vi "Meacurrent8341.vi"(8 "error in":errorcluster caption="错误输入", 10 "测试类型":u16(ring) items=["DCV", "ACV", "DCI", "ACI", "OHM", "RST", "CAP", "FRQ", "AUTO"], 11 "VISA资源名称":refnum<visa-resource-name>="COM1") -> (0 "错误输出":errorcluster, 2 "数值":dbl format="%#_3g", 3 "响应":string)   [LabVIEW 2013]
uses:
  C:/Program Files/National Instruments/LabVIEW 2013/examples/Instrument IO/Serial/support/Serial - Settings.ctl
  <vilib>/Instr/_visa.llb/VISA Flush IO Buffer Mask.ctl
  <vilib>/Instr/_visa.llb/VISA Configure Serial Port (Instr).vi
panel:
  in  "串口设置":T1={"波特率"=9600, "数据比特"=8, "奇偶"=enum."None", "停止位"=10, "流控制"=0} {"流控制" items=["无"=0, "XON/XOFF"=1, "RTS/CTS"=2, "DTR/DSR"=4]; "停止位" items=["1.0"=10, "1.5"=15, "2.0"=20]; "数据比特" min=5 max=8 step=1; "波特率" items=["75"=75, "110"=110, "134"=134, "150"=150, "300"=300, "600"=600, "1200"=1200, "1800"=1800, "2400"=2400, "4800"=4800, "7200"=7200, "9600"=9600, "14400"=14400, "19200"=19200, "28800"=28800, "38400"=38400, "56000"=56000, "57600"=57600, "115200"=115200, "128000"=128000, "230400"=230400]}
  in  "读取前延时(ms)":u32=200
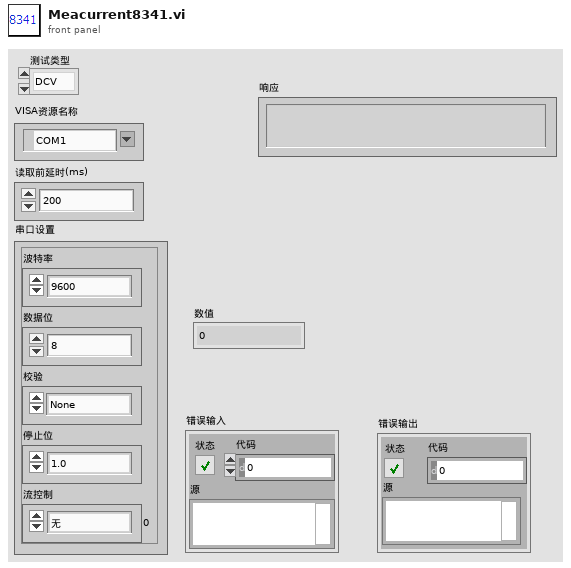
[diagram p1: front panel]
types:
  T1 = typedef "Serial - Settings.ctl" = cluster{"波特率":u32, "数据比特":u16, "奇偶":enum16{"None", "Odd", "Even", "Mark", "Space"}, "停止位":u16, "流控制":u16}
  T2 = typedef "VISA Flush IO Buffer Mask.ctl" = u16
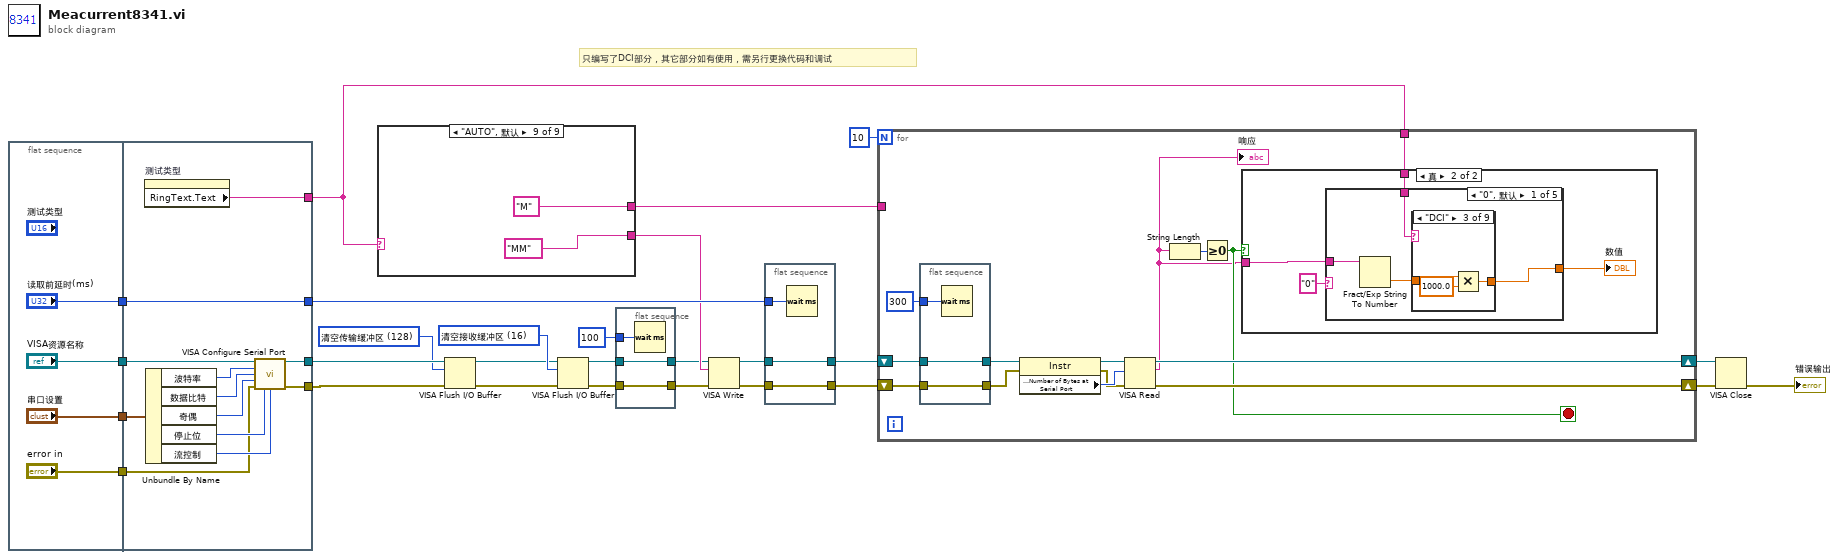
[diagram p0: block diagram]
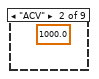
[diagram p4: hidden frame]
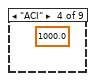
[diagram p5: hidden frame]
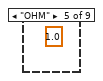
[diagram p6: hidden frame]
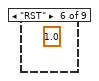
[diagram p7: hidden frame]
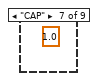
[diagram p8: hidden frame]
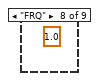
[diagram p9: hidden frame]
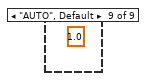
[diagram p10: hidden frame]
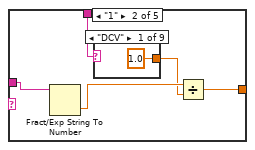
[diagram p11: hidden frame]
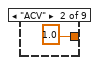
[diagram p12: hidden frame]
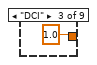
[diagram p13: hidden frame]
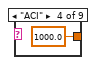
[diagram p14: hidden frame]
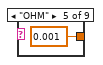
[diagram p15: hidden frame]
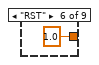
[diagram p16: hidden frame]
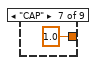
[diagram p17: hidden frame]
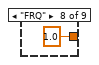
[diagram p18: hidden frame]
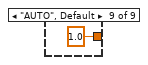
[diagram p19: hidden frame]
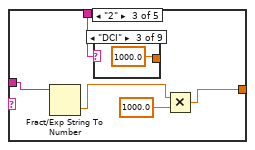
[diagram p20: hidden frame]
diagram:
  w7 = T2 128 items=["清空接收缓冲区"=16, "向设备写入传输缓冲区"=32, "清空接收缓冲区（无I/O）"=64, "清空传输缓冲区"=128] ("Mask")
  w16 = T2 16 items=["清空接收缓冲区"=16, "向设备写入传输缓冲区"=32, "清空接收缓冲区（无I/O）"=64, "清空传输缓冲区"=128] ("Mask")
  # "只编写了DCI部分，其它部分如有使用，需另行更换代码和调试"
  n1 = flat-sequence {
    tunnel: ["VISA资源名称"] -> w15
    tunnel: ["读取前延时(ms)"] -> w14
    tunnel: ["串口设置"] -> w13
    tunnel: ["error in"] -> w1
    tunnel: [w43] -> w23
    tunnel: w15 -> [w36]
    tunnel: w14 -> [w43]
    tunnel: w13 -> [w37]
    tunnel: [w35] -> w12
    tunnel: [w34] -> w11
    tunnel: [w33] -> w10
    tunnel: w1 -> [w32]
    frame #0 {
    }
    frame #1 {
      n2 = property on="测试类型" class="Ring (严格)"() -> ("RingText.Text"=w33:string)  [unwired: 2 in, 2 out]
      n3 = Unbundle By Name(w37) -> ("波特率"=w38:u32, "数据比特"=w39:u16, "奇偶"=w40:enum16{"None", "Odd", "Even", "Mark", "Space"}, "停止位"=w41:u16, "流控制"=w42:u16)
      n4 = call-poly "VISA Configure Serial Port"("VISA resource name"=w36, "baud rate (9600)"=w38, "data bits (8)"=w39, "parity (0:none)"=w40, "error in (no error)"=w32, "stop bits (10: 1 bit)"=w41, "flow control (0:none)"=w42) -> ("VISA resource name out"=w35:refnum<visa-resource-name>, "error out"=w34:errorcluster)  [unwired: 2 in, 5 out]
    }
  }
  n5 = case shown="\"AUTO\", 默认" w10 {
    tunnel: ["MEAS:VOLT:DC? 50e\n" "MEAS:VOLT:AC? 50e\n" "MEAS:CURR:DC? 5e\n" "MEAS:CURR:AC? 5e\n" "EE" ("Command") "FF" ("Command") "GG" ("Command") "HH" ("Command") "MM" ("Command")] -> w22
    tunnel: ["0" ("Command") "1" ("Command") "3" ("Command") "4" ("Command") "6" ("Command") "F" ("Command") "7" ("Command") "8" ("Command") "M" ("Command")] -> w21
    frame "DCV" {
      n6 = local write "数值"(0.0 ("数值")) -> ()
    }
    frame "ACV" {
      n7 = local write "数值"(0.0 ("数值")) -> ()
    }
    frame "DCI" {
      n8 = local write "数值"(0.0 ("数值")) -> ()
    }
    frame "ACI" {
    }
    frame "OHM" {
    }
    frame "RST" {
    }
    frame "CAP" {
    }
    frame "FRQ" {
    }
    frame "AUTO", Default {
    }
  }
  n9 = VISA Flush I/O Buffer(VISA resource name=w12, mask (16)=w7, error in (no error)=w11) -> (VISA resource name out=w9:refnum<visa-resource-name>, error out=w8:errorcluster)
  n10 = VISA Flush I/O Buffer(VISA resource name=w9, mask (16)=w16, error in (no error)=w8) -> (VISA resource name out=w6:refnum<visa-resource-name>, error out=w3:errorcluster)
  n11 = flat-sequence {
    tunnel: w6 -> [w67]
    tunnel: [w67] -> w5
    tunnel: [w66] -> w4
    tunnel: w3 -> [w66]
    tunnel: 100 -> [w65]
    frame #0 {
      n12 = Wait (ms)(milliseconds to wait=w65) -> ()  [unwired: 1 out]
    }
  }
  n13 = VISA Write(VISA resource name=w5, write buffer=w22, error in (no error)=w4) -> (VISA resource name out=w18:refnum<visa-resource-name>, error out=w17:errorcluster)  [unwired: 1 out]
  n14 = flat-sequence {
    tunnel: [w68] -> w25
    tunnel: [w69] -> w24
    tunnel: w23 -> [w70]
    tunnel: w18 -> [w69]
    tunnel: w17 -> [w68]
    frame #0 {
      n15 = Wait (ms)(milliseconds to wait=w70) -> ()  [unwired: 1 out]
    }
  }
  n16 = for {
    N: 10 -> [_]
    tunnel: w21 -> [_]
    tunnel: w10 -> [w81]
    shift-right: [w83] -> w26
    shift-left: w24 -> [w80]
    shift-right: [w84] -> w27
    shift-left: w25 -> [w78]
    stop <- w75 stop-if-true
    n17 = flat-sequence {
      tunnel: w78 -> [w86]
      tunnel: [w86] -> w77
      tunnel: w80 -> [w85]
      tunnel: [w85] -> w79
      tunnel: u32 300 ("读取前延时(ms)") -> [w87]
      frame #0 {
        n18 = Wait (ms)(milliseconds to wait=w87) -> ()  [unwired: 1 out]
      }
    }
    n19 = property class="Instr"(reference=w79, error in=w77) -> (reference out=w74:refnum<visa-resource-name>, error out=w73:errorcluster, "Serial Settings:Number of Bytes at Serial Port"=w82:u32)
    n20 = VISA Read(VISA resource name=w74, byte count=w82, error in (no error)=w73) -> (VISA resource name out=w83:refnum<visa-resource-name>, read buffer=w71:string, error out=w84:errorcluster)  [unwired: 1 out]
    "响应" <- w71
    n21 = String Length(string=w71) -> (length=w72:i32)
    n22 = Greater Or Equal To 0?(x=w72) -> (x >= 0?=w75:bool)
    n23 = case shown="真" w75 {
      tunnel: w71 -> [_ w88]
      tunnel: w81 -> [_ w91]
      frame False {
      }
      frame True {
        n24 = case shown="\"0\", 默认" "0" {
          tunnel: w88 -> [w95 w104 w118 w132 w146]
          tunnel: w91 -> [w94 w103 w117 w131 w145]
          tunnel: [w93 w100 w114 w128 w142] -> w90
          frame "0", Default {
            n25 = Fract/Exp String To Number(string=w95) -> (number=w92:dbl)  [unwired: 3 in, 1 out]
            n26 = case shown="\"DCI\"" w94 {
              tunnel: [w96 _ w97 _ _ _ _ _ _] -> w93
              tunnel: w92 -> [w96 _ w99 _ _ _ _ _ _]
              frame "DCV" {
              }
              frame "ACV" {
                (unwired) 1000.0
              }
              frame "DCI" {
                n27 = Multiply(x=w99, y=1000.0) -> (x*y=w97:dbl)
              }
              frame "ACI" {
                (unwired) 1000.0
              }
              frame "OHM" {
                (unwired) 1.0
              }
              frame "RST" {
                (unwired) 1.0
              }
              frame "CAP" {
                (unwired) 1.0
              }
              frame "FRQ" {
                (unwired) 1.0
              }
              frame "AUTO", Default {
                (unwired) 1.0
              }
            }
          }
          frame "1" {
            n28 = Fract/Exp String To Number(string=w104) -> (number=w102:dbl)  [unwired: 3 in, 1 out]
            n29 = case shown="\"DCV\"" w103 {
              tunnel: [1.0 1.0 1.0 1000.0 0.001 1.0 1.0 1.0 1.0] -> w101
              frame "DCV" {
              }
              frame "ACV" {
              }
              frame "DCI" {
              }
              frame "ACI" {
              }
              frame "OHM" {
              }
              frame "RST" {
              }
              frame "CAP" {
              }
              frame "FRQ" {
              }
              frame "AUTO", Default {
              }
            }
            n30 = Divide(x=w102, y=w101) -> (x/y=w100:dbl)
          }
          frame "2" {
            n31 = Fract/Exp String To Number(string=w118) -> (number=w116:dbl)  [unwired: 3 in, 1 out]
            n32 = case shown="\"DCI\"" w117 {
              tunnel: [1.0 1.0 1000.0 1000.0 0.001 1.0 1.0 1.0 1.0] -> _
              frame "DCV" {
              }
              frame "ACV" {
              }
              frame "DCI" {
              }
              frame "ACI" {
              }
              frame "OHM" {
              }
              frame "RST" {
              }
              frame "CAP" {
              }
              frame "FRQ" {
              }
              frame "AUTO", Default {
              }
            }
            n33 = Multiply(x=w116, y=1000.0) -> (x*y=w114:dbl)
          }
          frame "3" {
            n34 = Fract/Exp String To Number(string=w132) -> (number=w130:dbl)  [unwired: 3 in, 1 out]
            n35 = case shown="\"DCI\"" w131 {
              tunnel: [1.0 1.0 1000.0 1000.0 0.001 1.0 1.0 1.0 1.0] -> w129
              frame "DCV" {
              }
              frame "ACV" {
              }
              frame "DCI" {
              }
              frame "ACI" {
              }
              frame "OHM" {
              }
              frame "RST" {
              }
              frame "CAP" {
              }
              frame "FRQ" {
              }
              frame "AUTO", Default {
              }
            }
            n36 = Divide(x=w130, y=w129) -> (x/y=w128:dbl)
          }
          frame "4" {
            n37 = Fract/Exp String To Number(string=w146) -> (number=w144:dbl)  [unwired: 3 in, 1 out]
            n38 = case shown="\"DCI\"" w145 {
              tunnel: [1.0 1.0 1000.0 1000.0 1e-06 1.0 1.0 1.0 1.0] -> w143
              frame "DCV" {
              }
              frame "ACV" {
              }
              frame "DCI" {
              }
              frame "ACI" {
              }
              frame "OHM" {
              }
              frame "RST" {
              }
              frame "CAP" {
              }
              frame "FRQ" {
              }
              frame "AUTO", Default {
              }
            }
            n39 = Divide(x=w144, y=w143) -> (x/y=w142:dbl)
          }
        }
        "数值" <- w90
      }
    }
  }
  n40 = VISA Close(VISA resource name=w26, error in (no error)=w27) -> (error out=→"错误输出":errorcluster)
